vi "Record Fiducial.vi"(9 "CH index":i32, 10 "XYZ":dbl[](array[numeric]), 11 "input cluster":T1) -> (2 "All fiducials recorded":bool, 3 "output cluster":T1)   [LabVIEW 2021, in "Component Tray.lvclass"]
uses:
  Component Tray.lvclass
  Find Component.ctl
  Controller/Camera/Machine Vision.ctl
  Component Tray.lvclass/Component Tray.ctl
  Controller/Camera/Camera.lvclass
panel:
  out "XYZTheta":dbl[](array[numeric]) format="%.6g"
  out "CH1 XYZ":dbl[](array[numeric])
  out "Sensor ID Location":dbl[](array[numeric])
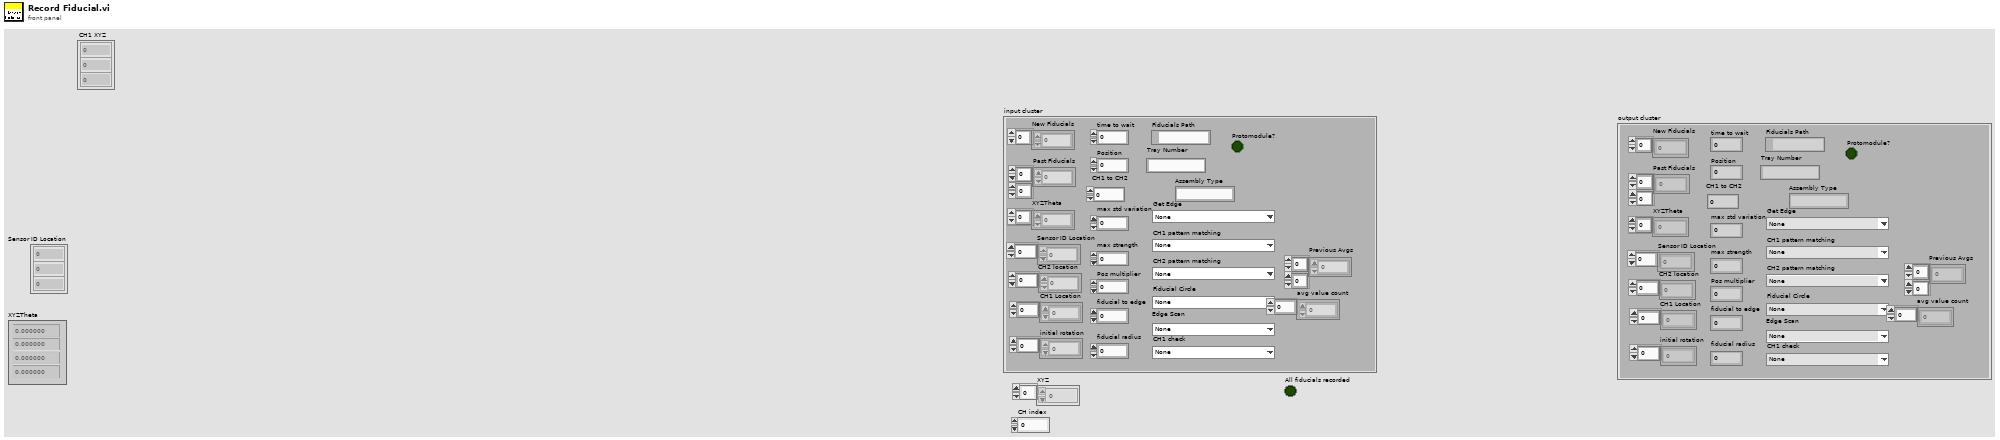
[diagram p1: front panel]
types:
  T1 = typedef "Component Tray.lvclass/Find Component.ctl" = cluster{"New Fiducials":dbl[], "Past Fiducials":dbl[][], "XYZTheta":dbl[], "Fiducials Path":path, "Position":i32, "CH1 Location":dbl[], "Sensor ID Location":dbl[], "initial rotation":dbl[], "CH2 location":dbl[], "max std variation":dbl, "max strength":dbl, "CH2 pattern matching":T2, "Fiducial Circle":T2, "Get Edge":T2, "Pos multiplier":dbl, "time to wait":u32, "fiducial to edge":dbl, "Protomodule?":bool, "Assembly Type":string, "CH1 to CH2":dbl, "Tray Number":string, "fiducial radius":dbl, "4 fiducials?":bool, "CH1 check":T2, "Edge Scan":T2, "CH1 pattern matching":T2, "Sensor Thickness":dbl, "Previous Avgs":dbl[][], "avg value count":dbl[]}
  T2 = typedef "Camera.lvclass/Machine Vision.ctl" = enum16{"None", "Assembly Tray Circle", "Assembly Tray Fiducial", "Partial Hexaboard", "sensor edge init", "HB edge init", "sensor edge pos1", "sensor edge pos2", "HB edge pos1", "HB edge pos2", "Sensor CH1-2", "HB CH1", "HB CH2", "V3 Sensor Circle", "Hexaboard Circle", "sensor CH1 check", "HB CH1 check ", "sensor ID"}
  T3 = typedef "File Paths.ctl" = cluster{"Glue Pattern Folder":path, "Carrier Tray Folder":path, "Pick Up Tool Fixture Folder":path, "Components Folder":path, "Bellows Tool Offset.txt":path, "Pick Up Tool Offset.txt":path, "Dispense Tip Offset.txt":path, "Log Files":path, "Gantry Assembly Map.txt":path, "Syringe and offset map.txt":path, "Controllers Folder":path, "Local dbase config":path}
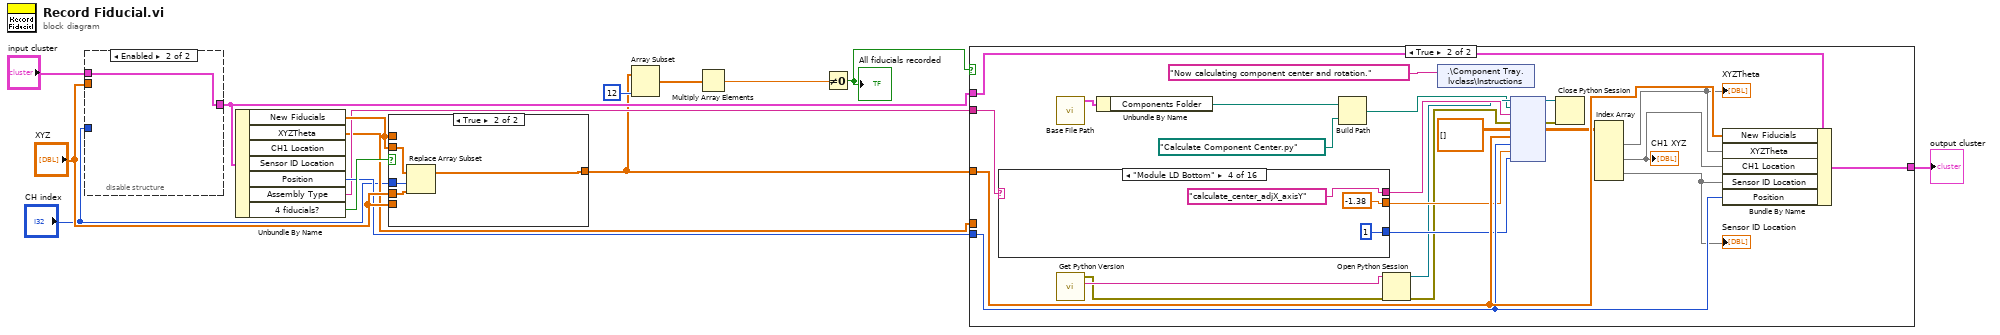
[diagram p0: block diagram]
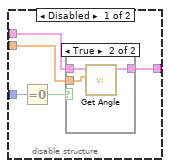
[diagram p2: hidden frame]
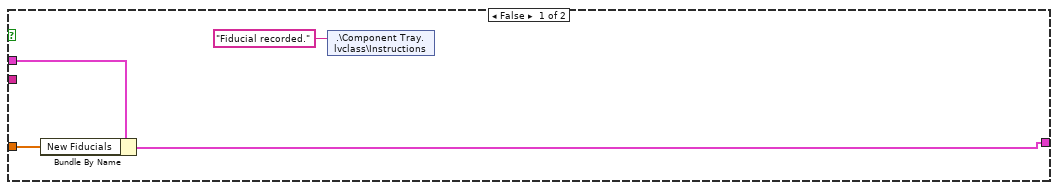
[diagram p4: hidden frame]
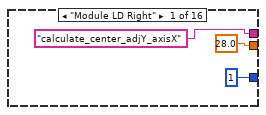
[diagram p5: hidden frame]
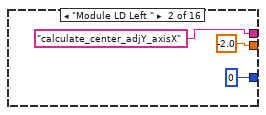
[diagram p6: hidden frame]
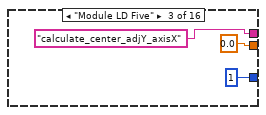
[diagram p7: hidden frame]
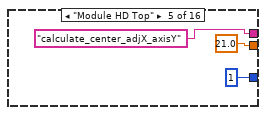
[diagram p8: hidden frame]
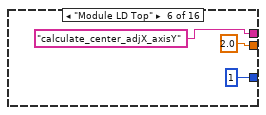
[diagram p9: hidden frame]
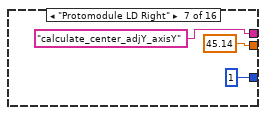
[diagram p10: hidden frame]
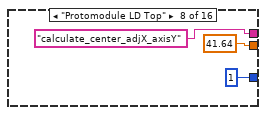
[diagram p11: hidden frame]
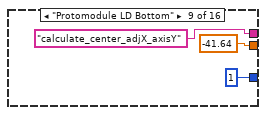
[diagram p12: hidden frame]
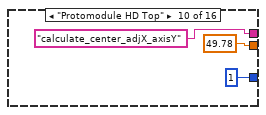
[diagram p13: hidden frame]
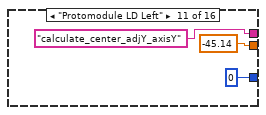
[diagram p14: hidden frame]
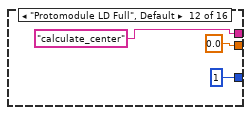
[diagram p15: hidden frame]
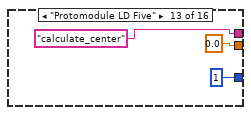
[diagram p16: hidden frame]
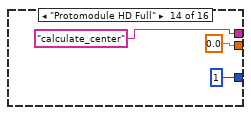
[diagram p17: hidden frame]
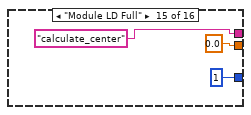
[diagram p18: hidden frame]
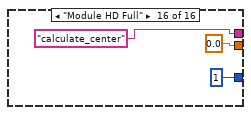
[diagram p19: hidden frame]
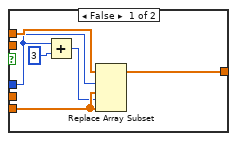
[diagram p20: hidden frame]
diagram:
  n1 = disable-structure shown="Enabled" {
    disable-tunnel: "input cluster" -> [w20 w25]
    disable-tunnel: "XYZ" -> [w19 _]
    disable-tunnel: [w18 w25] -> w4
    disable-tunnel: "CH index" -> [w17 _]
    frame Disabled {
      n2 = Equal To 0?(x=w17) -> (x = 0?=w16:bool)
      n3 = case shown="True" w16 {
        tunnel: w20 -> [w21 w24]
        tunnel: [w21 w23] -> w18
        tunnel: w19 -> [_ w22]
        frame False {
        }
        frame True {
          n4 = call "Get Angle.vi"("array"=w22, "input cluster"=w24) -> ("output cluster"=w23:T1)  [unwired: 8 in, 1 out]
        }
      }
    }
    frame Enabled {
    }
  }
  n5 = Unbundle By Name(w4) -> ("New Fiducials"=w15:dbl[], "XYZTheta"=w5:dbl[], "Position"=w7:i32, "Assembly Type"=w6:string, "4 fiducials?"=w14:bool)  [unwired: 2 out]
  n6 = case shown="True" w14 {
    tunnel: w15 -> [w31 _]
    tunnel: "XYZ" -> [w30 _]
    tunnel: [w27 w32] -> w2
    tunnel: w15 -> [_ w35]
    tunnel: "XYZ" -> [_ w34]
    tunnel: "CH index" -> [w26 w33]
    frame False {
      n7 = Add(x=w26, y=3) -> (x+y=w28:i32)
      n8 = Replace Array Subset "Replace Array Subset"(array=w31, new element #1=w30, index #1=w26, new element #2=w30, index #2=w28) -> (w27:dbl[])
    }
    frame True {
      n9 = Replace Array Subset "Replace Array Subset"(array=w35, new element=w34, index=w33) -> (w32:dbl[])
    }
  }
  n10 = Array Subset "Array Subset"(array=w2, length=12) -> (w9:dbl[])  [unwired: 1 in]
  n11 = Multiply Array Elements(1:w9) -> (0:w10:dbl)
  n12 = Not Equal To 0?(x=w10) -> (x != 0?=w8:bool)
  "All fiducials recorded" <- w8
  n13 = case shown="True" w8 {
    tunnel: w2 -> [w38 w63]
    tunnel: w5 -> [_ _]
    tunnel: w7 -> [_ w62]
    tunnel: w4 -> [w39 w61]
    tunnel: [w37 w60] -> w1
    tunnel: w6 -> [_ w59]
    frame False {
      n14 = Bundle By Name(cluster=w39, "New Fiducials"=w38) -> (w37:T1)
      n15 = shared-variable ".\\Component Tray.lvclass\\Instructions"("Fiducial recorded." ("Instructions")) -> ()  [unwired: 1 in, 1 out]
    }
    frame True {
      n16 = case shown="\"Module LD Bottom\"" w59 {
        tunnel: ["calculate_center_adjY_axisX" ("function name") "calculate_center_adjY_axisX" ("function name") "calculate_center_adjY_axisX" ("function name") "calculate_center_adjX_axisY" ("function name") "calculate_center_adjX_axisY" ("function name") "calculate_center_adjX_axisY" ("function name") "calculate_center_adjY_axisY" ("function name") "calculate_center_adjX_axisY" ("function name") "calculate_center_adjX_axisY" ("function name") "calculate_center_adjX_axisY" ("function name") "calculate_center_adjY_axisY" ("function name") "calculate_center" ("function name") "calculate_center" ("function name") "calculate_center" ("function name") "calculate_center" ("function name") "calculate_center" ("function name")] -> w55
        tunnel: [28.0 -2.0 0.0 -1.38 21.0 2.0 45.14 41.64 -41.64 49.78 -45.14 0.0 0.0 0.0 0.0 0.0] -> w54
        tunnel: [1 0 1 1 1 1 1 1 1 1 0 1 1 1 1 1] -> w53
        frame "Module LD Right" {
        }
        frame "Module LD Left " {
        }
        frame "Module LD Five" {
        }
        frame "Module LD Bottom" {
        }
        frame "Module HD Top" {
        }
        frame "Module LD Top" {
        }
        frame "Protomodule LD Right" {
        }
        frame "Protomodule LD Top" {
        }
        frame "Protomodule LD Bottom" {
        }
        frame "Protomodule HD Top" {
        }
        frame "Protomodule LD Left" {
        }
        frame "Protomodule LD Full", Default {
        }
        frame "Protomodule LD Five" {
        }
        frame "Protomodule HD Full" {
        }
        frame "Module LD Full" {
        }
        frame "Module HD Full" {
        }
      }
      n17 = call "Base File Path.vi"() -> ("Paths Out"=w48:T3)  [unwired: 11 in]
      n18 = call "Get Python Version.vi"() -> ("Python Version"=w42:string, "error out"=w41:errorcluster)  [unwired: 10 in]
      n19 = Unbundle By Name(w48) -> ("Components Folder"=w46:path)
      n20 = Build Path(base path=w46, name or relative path=path "Calculate Component Center.py") -> (appended path=w45:path)
      n21 = Open Python Session(python version=w42, 3:w41) -> (session out=w52:refnum<k35>, error out=w50:errorcluster)  [unwired: 1 in]
      n22 = shared-variable ".\\Component Tray.lvclass\\Instructions"("Now calculating component center and rotation." ("Instructions")) -> ()  [unwired: 1 in, 1 out]
      n23 = node(w52, w45, w55, w50, dbl[][] [], w63, w62, w54, w53) -> (w51:refnum<k35>, w49:errorcluster, w43:dbl[][])  [unwired: 4 in, 2 out]
      n24 = Close Python Session(session in=w51, error in=w49) -> ()  [unwired: 1 out]
      n25 = Index Array(array=w43) -> (element #1=w56:dbl[], element #2=w57:dbl[], element #3=w58:dbl[])  [unwired: 6 in]
      "XYZTheta" <- w56
      "CH1 XYZ" <- w57
      "Sensor ID Location" <- w58
      n26 = Bundle By Name(cluster=w61, "New Fiducials"=w63, "XYZTheta"=w56, "CH1 Location"=w57, "Sensor ID Location"=w58, "Position"=w62) -> (w60:T1)
    }
  }
  "output cluster" <- w1
